vi "PLC.Connect.vi"(8 "error in (no error)":errorcluster, 11 "Data":T1={"Status"={"Idx"=0, "ConnRef"=0, "State"=enum."Off", "LiveBitTimer"=timestamp(0 s since 1904-01-01)}, "Sets"={"Enable"=FALSE, "IP"="", "Rack"=0, "Slot"=0, "LifeBitTimer_s"=0.0, "DataBlockAddr_PCStatus"=0, "DataBlockAddr_PLCStatus"=1, "DataBlockAddr_PLCNewData"=[], "DataBlockSize_PLCNewData"=[], "DataBlockAddr_PLCChangeOver"=[], "DataBlockSize_PLCChangeOver"=[], "DataBlockAddr_PCChangeOver"=[], "DataBlockAddr_PLCCheckStatus"=[], "DataBlockSize_PLCCheckStatus"=[], "DataBlockAddr_PCCheckStatus"=[], "System"=""}, "PCstatus"={"General"={"LifeBit"=FALSE, "DbRun"=FALSE}, "Stations"=[]}, "PLCstatus"={"General"={"LifeBit"=FALSE}, "Stations"=[]}}) -> (0 "error out":errorcluster, 3 "Data out":T1={"Status"={"Idx"=0, "ConnRef"=0, "State"=enum."Off", "LiveBitTimer"=timestamp(0 s since 1904-01-01)}, "Sets"={"Enable"=FALSE, "IP"="", "Rack"=0, "Slot"=0, "LifeBitTimer_s"=0.0, "DataBlockAddr_PCStatus"=0, "DataBlockAddr_PLCStatus"=1, "DataBlockAddr_PLCNewData"=[], "DataBlockSize_PLCNewData"=[], "DataBlockAddr_PLCChangeOver"=[], "DataBlockSize_PLCChangeOver"=[], "DataBlockAddr_PCChangeOver"=[], "DataBlockAddr_PLCCheckStatus"=[], "DataBlockSize_PLCCheckStatus"=[], "DataBlockAddr_PCCheckStatus"=[], "System"=""}, "PCstatus"={"General"={"LifeBit"=FALSE, "DbRun"=FALSE}, "Stations"=[]}, "PLCstatus"={"General"={"LifeBit"=FALSE}, "Stations"=[]}})   [LabVIEW 2016]
doc: "Connect to PLC\n\nWabco 2017 All right reserved\nAuthor: maciej.szupienko@wabco-auto.com"
uses:
  PLC.Data.ctl
  PLC.Data.Status.ctl
  PLC.State.ctl
  PLC.Data.Sets.ctl
  LowLevel/PLC.DataBlock.PCstatus.ctl
  LowLevel/PLC.DataBlock.PCstatus.General.ctl
  LowLevel/PLC.DataBlock.PCstatus.Station.ctl
  LowLevel/PLC.DataBlock.PLCstatus.ctl
  LowLevel/PLC.DataBlock.PLCstatus.General.ctl
  LowLevel/PLC.DataBlock.PLCstatus.Station.ctl
  Snap7/lib/Snap7.lvlib
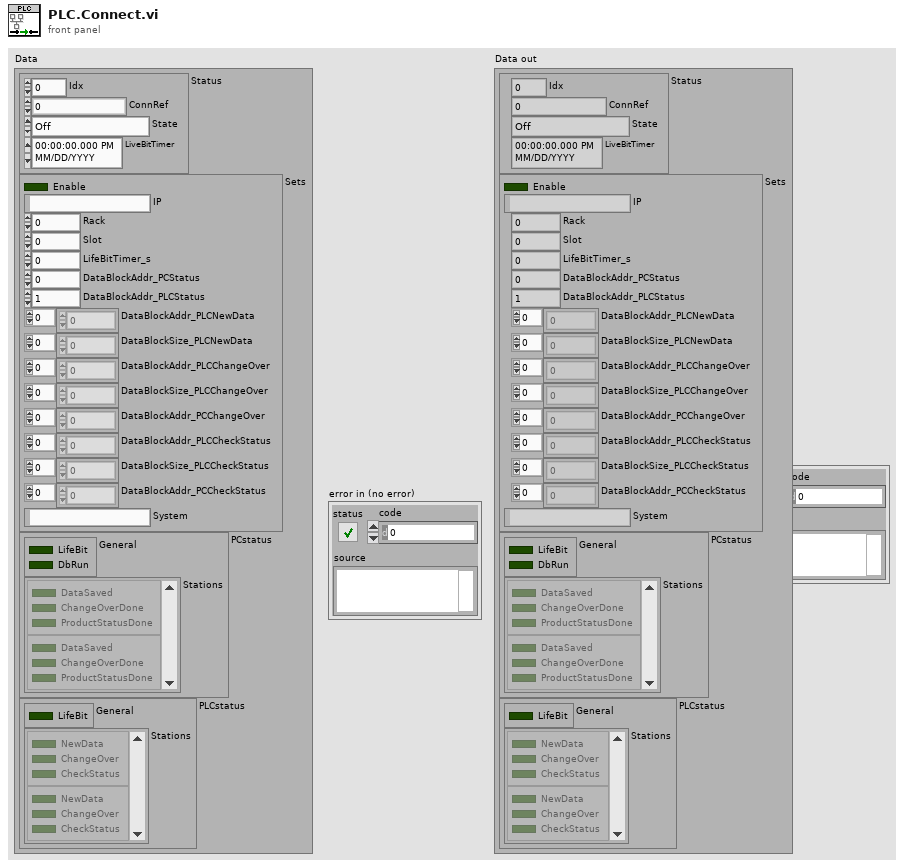
[diagram p1: front panel]
types:
  T1 = typedef "PLC.Data.ctl" = cluster{"Status":T2, "Sets":T4, "PCstatus":T5, "PLCstatus":T8}
  T2 = typedef "PLC.Data.Status.ctl" = cluster{"Idx":i32, "ConnRef":u64, "State":T3, "LiveBitTimer":timestamp}
  T3 = typedef "PLC.State.ctl" = enum32{"Off", "Error", "Idle", "Run"}
  T4 = typedef "PLC.Data.Sets.ctl" = cluster{"Enable":bool, "IP":string, "Rack":i32, "Slot":i32, "LifeBitTimer_s":dbl, "DataBlockAddr_PCStatus":i32, "DataBlockAddr_PLCStatus":i32, "DataBlockAddr_PLCNewData":i32[], "DataBlockSize_PLCNewData":i32[], "DataBlockAddr_PLCChangeOver":i32[], "DataBlockSize_PLCChangeOver":i32[], "DataBlockAddr_PCChangeOver":i32[], "DataBlockAddr_PLCCheckStatus":i32[], "DataBlockSize_PLCCheckStatus":i32[], "DataBlockAddr_PCCheckStatus":i32[], "System":string}
  T5 = typedef "PLC.DataBlock.PCstatus.ctl" = cluster{"General":T6, "Stations":T7[]}
  T6 = typedef "PLC.DataBlock.PCstatus.General.ctl" = cluster{"LifeBit":bool, "DbRun":bool}
  T7 = typedef "PLC.DataBlock.PCstatus.Station.ctl" = cluster{"DataSaved":bool, "ChangeOverDone":bool, "ProductStatusDone":bool}
  T8 = typedef "PLC.DataBlock.PLCstatus.ctl" = cluster{"General":T9, "Stations":T10[]}
  T9 = typedef "PLC.DataBlock.PLCstatus.General.ctl" = cluster{"LifeBit":bool}
  T10 = typedef "PLC.DataBlock.PLCstatus.Station.ctl" = cluster{"NewData":bool, "ChangeOver":bool, "CheckStatus":bool}
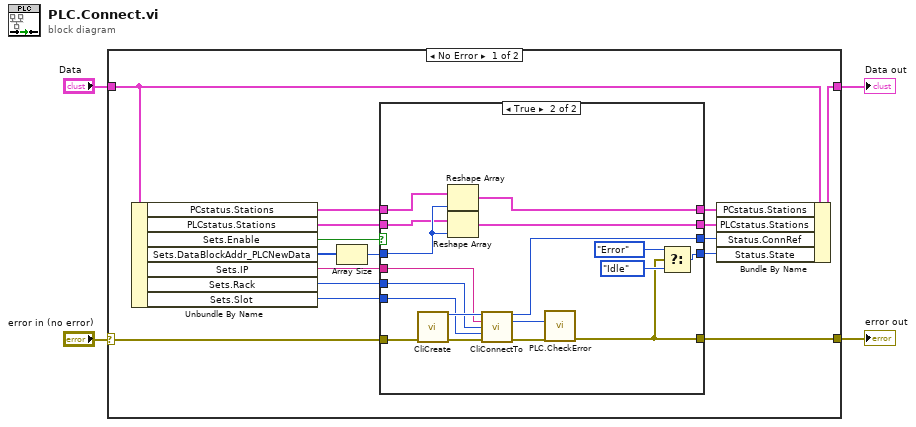
[diagram p0: block diagram]
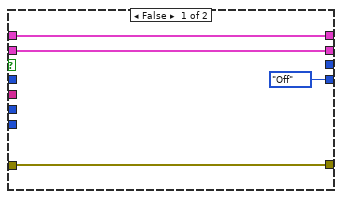
[diagram p2: hidden frame]
diagram:
  n1 = case shown="No Error" "error in (no error)" {
    selector: "error in (no error)" -> [w17 w44]
    tunnel: [w12 w44] -> w4
    tunnel: "Data" -> [w20 w43]
    tunnel: [w19 w43] -> w1
    frame No Error {
      n2 = Unbundle By Name(w20) -> ("PCstatus.Stations"=w10:T7[], "PLCstatus.Stations"=w9:T10[], "Sets.Enable"=w11:bool, "Sets.DataBlockAddr_PLCNewData"=w8:i32[], "Sets.IP"=w15:string, "Sets.Rack"=w14:i32, "Sets.Slot"=w13:i32)
      n3 = Array Size(array=w8) -> (size(s)=w5:i32)
      n4 = case shown="True" w11 {
        tunnel: [PLC.State."Off" ("Status.Action") w40] -> w18
        tunnel: w17 -> [w23 w39]
        tunnel: [_ w37] -> w16
        tunnel: w15 -> [_ w35]
        tunnel: w14 -> [_ w34]
        tunnel: w13 -> [_ w33]
        tunnel: [w23 w31] -> w12
        tunnel: w10 -> [w22 w26]
        tunnel: w9 -> [w21 w27]
        tunnel: w5 -> [_ w28]
        tunnel: [w22 w25] -> w7
        tunnel: [w21 w29] -> w6
        frame False {
        }
        frame True {
          n5 = call "CliCreate.vi"("error in (no error)"=w39) -> ("ref out"=w36:u64, "error out"=w38:errorcluster)  [unwired: 13 in]
          n6 = Reshape Array(w26, w28) -> (w25:T7[])
          n7 = Reshape Array(w27, w28) -> (w29:T10[])
          n8 = call "CliConnectTo.vi"("ref in"=w36, "Address"=w35, "Rack"=w34, "Slot"=w33, "error in (no error)"=w38) -> ("ref out"=w37:u64, "Result"=w30:i32, "error out"=w32:errorcluster)  [unwired: 8 in]
          n9 = call "PLC.CheckError.vi"("error in (no error)"=w32, "Result"=w30) -> ("error out"=w31:errorcluster)  [unwired: 9 in]
          n10 = Select(t=PLC.State."Error" ("Status.Action"), s=w31, f=PLC.State."Idle" ("Status.Action")) -> (s? t:f=w40:T3)
        }
      }
      n11 = Bundle By Name(cluster=w20, "PCstatus.Stations"=w7, "PLCstatus.Stations"=w6, "Status.ConnRef"=w16, "Status.State"=w18) -> (w19:T1)
    }
    frame Error {
    }
  }
  "error out" <- w4
  "Data out" <- w1
